vi "motion test.vi"() -> ()   [LabVIEW 2020]
uses:
  Classes/Controller/Controller.lvclass
  Classes/Controller/Motion/Motion.lvclass
panel:
  in  "stop":bool
  in  "Go":bool
  in  "XY Input":dbl[](array[numeric])
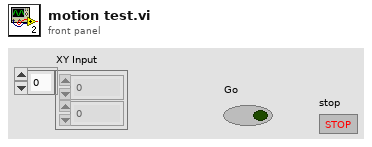
[diagram p1: front panel]
types:
  T1 = typedef "Controller.lvclass/Controllers.ctl" = cluster{"I-O.lvclass":refnum<class "I-O.lvclass">, "Dispenser.lvclass":refnum<class "Dispenser.lvclass">, "Gantry":refnum<k24>}
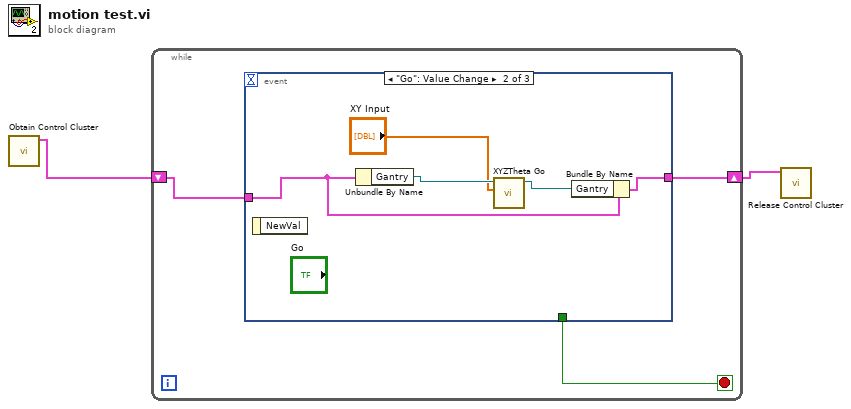
[diagram p0: block diagram]
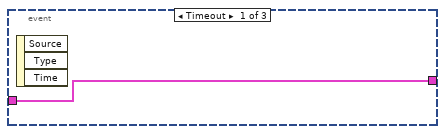
[diagram p2: hidden frame]
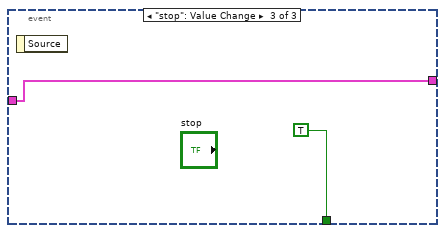
[diagram p3: hidden frame]
diagram:
  n1 = call "Obtain Control Cluster.vi"() -> ("Control Out"=w2:T1)  [unwired: 11 in]
  n2 = while {
    shift-right: [w3] -> w1
    shift-left: w2 -> [w4]
    stop <- w5 stop-if-true
    n3 = event shown="[1] \"Go\": Value Change" {
      selector: _ -> [_ _ _]
      dyn-events: _ -> [_ _ _]
      timeout: _ -> [_ _ _]
      tunnel: [_ _ TRUE] -> w5
      tunnel: w4 -> [w6 w9 w12]
      tunnel: [w6 w7 w12] -> w3
      event Timeout {
        n4 = event-data() -> ()  [unwired: 1 in, 3 out]
      }
      event "Go": Value Change {
        n5 = event-data() -> ()  [unwired: 1 in, 1 out]
        n6 = Unbundle By Name(w9) -> ("Gantry"=w11:refnum<k24>)
        n7 = call "XYZTheta Go.vi"("XYZTheta In"="XY Input", "Gantry 2"=w11) -> ("Gantry 3"=w8:refnum<k24>)  [unwired: 7 in, 2 out]
        n8 = Bundle By Name(cluster=w9, "Gantry"=w8) -> (w7:T1)
      }
      event "stop": Value Change {
        n9 = event-data() -> ()  [unwired: 1 in, 1 out]
      }
    }
  }
  n10 = call "Release Control Cluster.vi"("output cluster"=w1) -> ()  [unwired: 11 in]
